vi "DAQ_Pressure_Task.vi"(8 "error in":errorcluster) -> (0 "error out":errorcluster, 3 "task out":refnum<k21>)   [LabVIEW 2015]
uses:
  <vilib>/DAQmx/configure/timing.llb/DAQmx Timing (Sample Clock).vi
  <vilib>/DAQmx/create/channels.llb/DAQmx Create Channel (AI-Current-Basic).vi
  <vilib>/DAQmx/create/channels.llb/DAQmx Create Channel (TEDS-AI-Current-Basic).vi
  <vilib>/DAQmx/create/channels.llb/DAQmx Create Channel (TEDS-AI-Voltage-Basic).vi
  <vilib>/DAQmx/create/channels.llb/DAQmx Create Channel (AI-Voltage-Basic).vi
  <resource>/objmgr/daqmx.rc
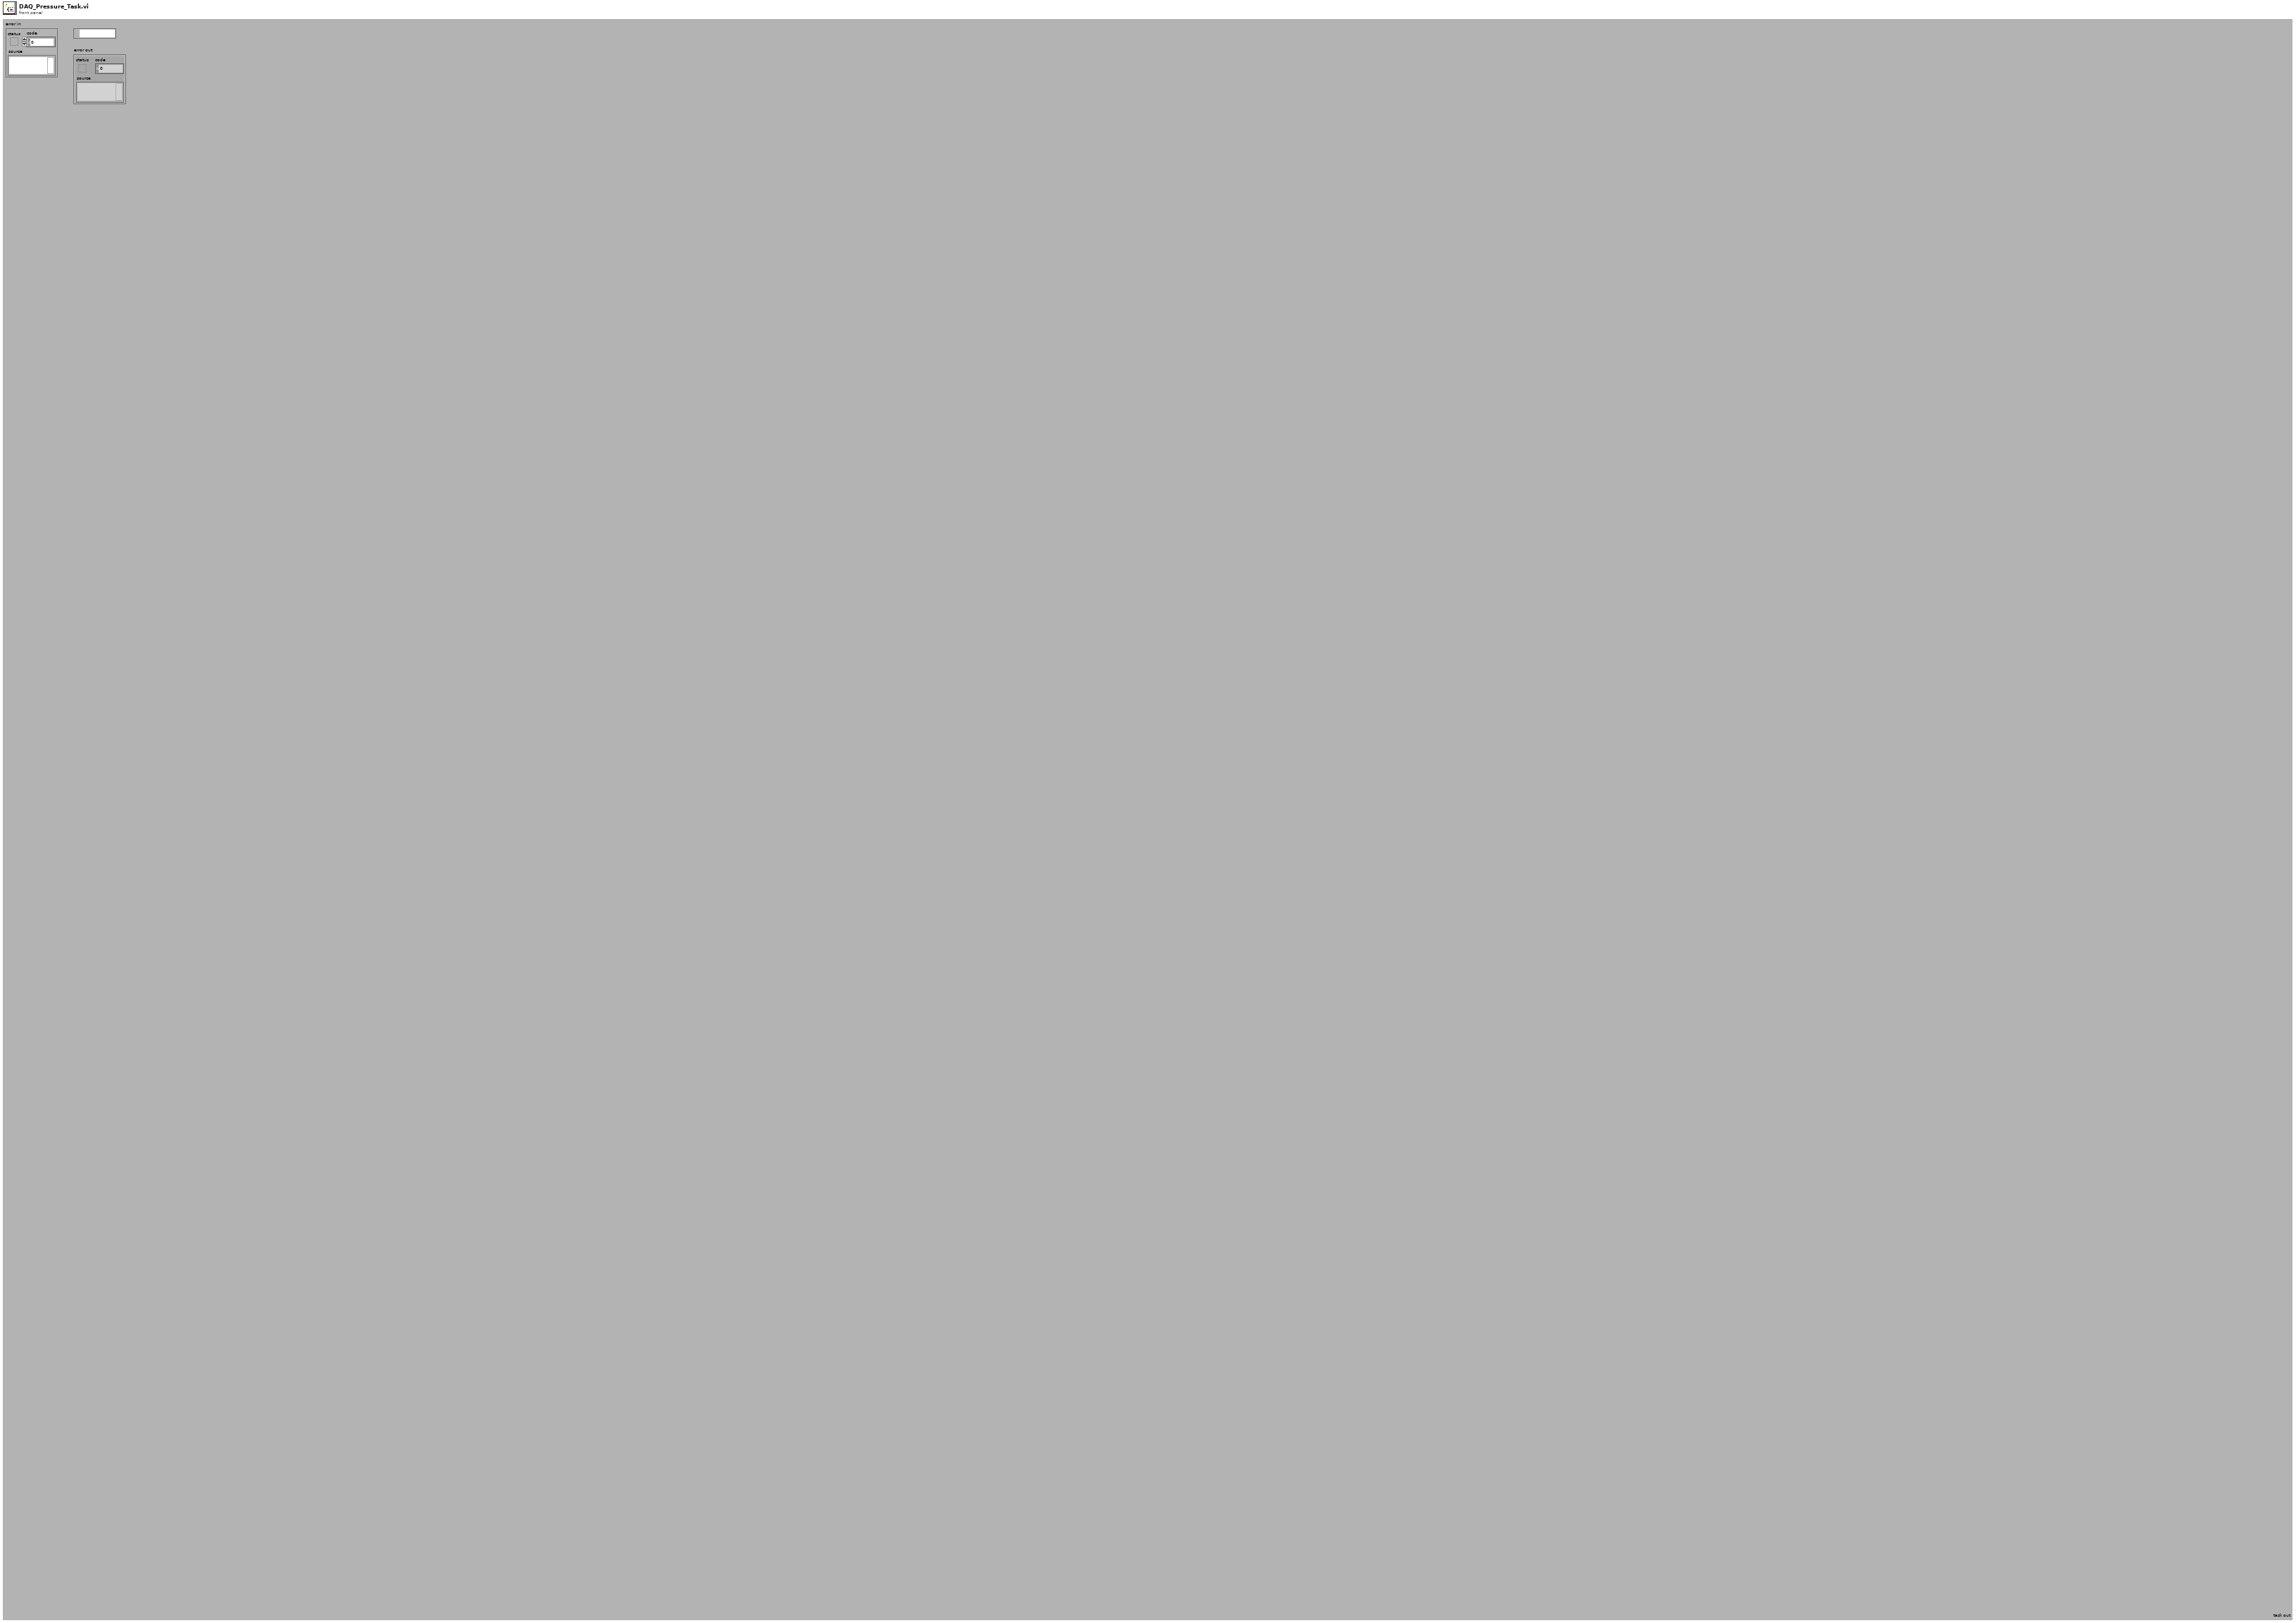
[diagram p1: front panel]
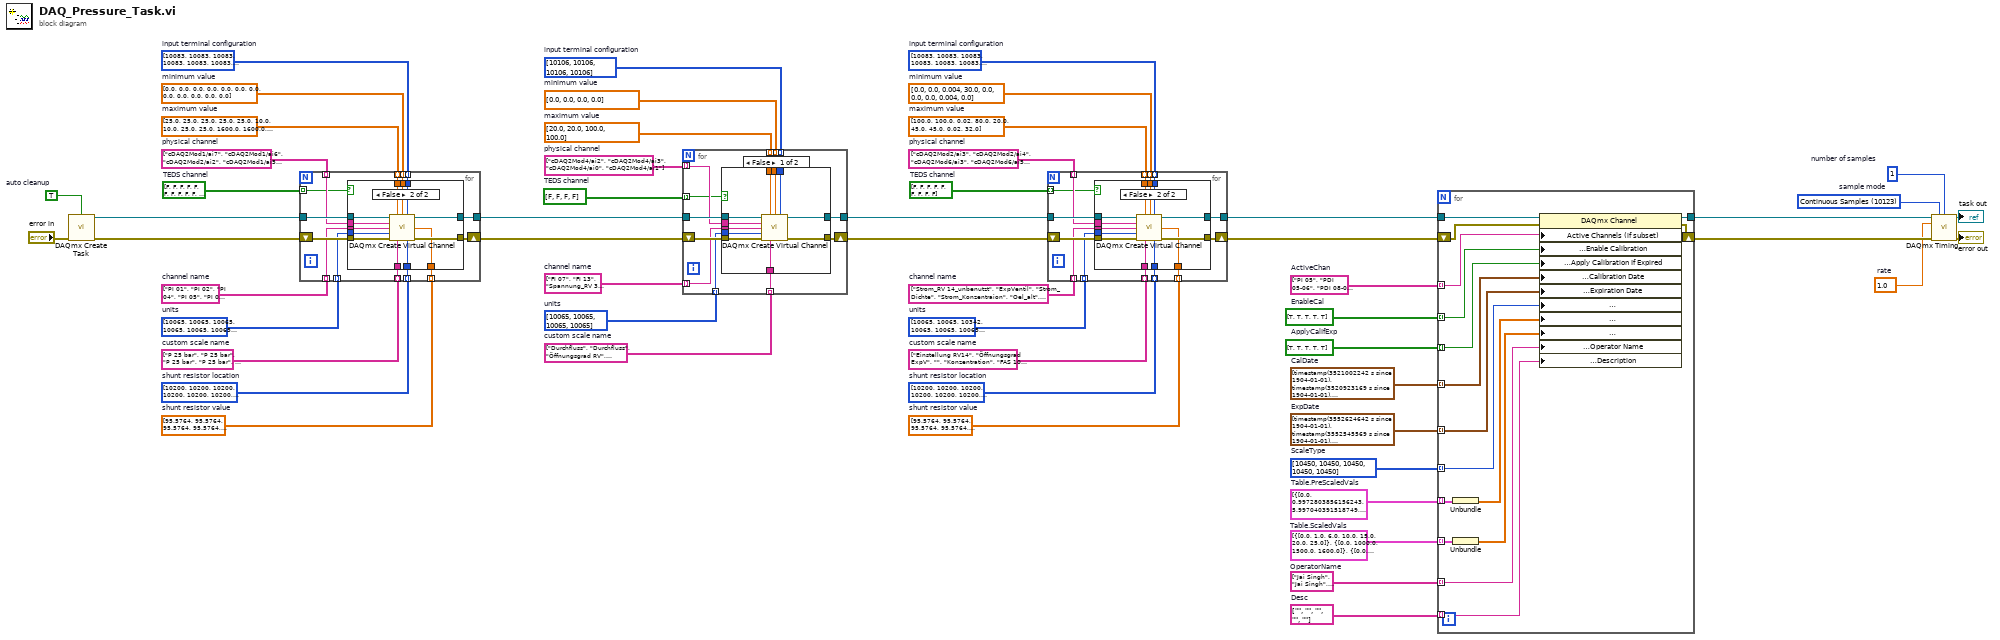
[diagram p0: block diagram]
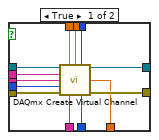
[diagram p2: hidden frame]
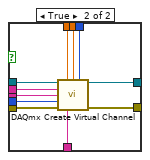
[diagram p3: hidden frame]
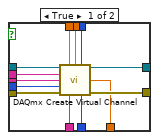
[diagram p4: hidden frame]
diagram:
  w1 = 10123 items=["Finite Samples"=10178, "Continuous Samples"=10123, "Hardware Timed Single Point"=12522]  # sample mode
  w2 = 1  # number of samples
  w3 = 1.0  # rate
  w7 = cluster{dbl[]}[] [{[0.0, 1.0, 6.0, 10.0, 15.0, 20.0, 25.0]}, {[0.0, 1000.0, 1500.0, 1600.0]}, {[0.0, 1000.0, 1500.0, 1600.0]}, {[0.0, 0.86, 1.21, 1.86, 3.1, 4.77, 6.65, 7.29, 8.84, 11.07, 13.51, 15.33, 20.0]}, {[0.004, 2.2, 3.42, 4.08, 7.7, 10.52, 12.92, 14.78, 20.74, 25.09, 26.53]}]  # Table.ScaledVals
  w8 = cluster{dbl[]}[] [{[0.0, 0.9972803856156243, 5.997040391518749, 10.015593347959374, 15.013742730296872, 20.021790629837497, 25.0]}, {[3.151240878800008, 1003.6394992132, 1504.2596451523, 1600.0]}, {[4.835925838111832, 998.5875410040248, 1496.213154230559, 1600.0]}, {[0.0, 0.6762841877287502, 1.0186559843750003, 1.6656615945525002, 2.9056125350500004, 4.562310075791251, 6.450162397260001, 7.0884341397075, 8.617806368865, 10.8448007925575, 13.286177970001251, 15.10389574293875, 20.0]}, {[0.004, 2.57, 3.6, 4.11, 7.72, 10.55, 13.02, 14.91, 21.22, 25.78, 26.53]}]  # Table.PreScaledVals
  w9 = string[] ["", "", "", "", ""]  # Desc
  w10 = string[] ["Jai Singh", "Jai Singh", "Jai Singh", "Tobi", "Max"]  # OperatorName
  w11 = timestamp[] [timestamp(3521002242.44 s since 1904-01-01), timestamp(3520923169.435 s since 1904-01-01), timestamp(3520930491.14 s since 1904-01-01), timestamp(3519973936.268 s since 1904-01-01), timestamp(3537180162.561 s since 1904-01-01)]  # CalDate
  w15 = bool[] [TRUE, TRUE, TRUE, TRUE, TRUE]  # EnableCal
  w14 = bool[] [TRUE, TRUE, TRUE, TRUE, TRUE]  # ApplyCalIfExp
  w13 = timestamp[] [timestamp(3552624642 s since 1904-01-01), timestamp(3552545569 s since 1904-01-01), timestamp(3552552891 s since 1904-01-01), timestamp(3551596336 s since 1904-01-01), timestamp(3568802563 s since 1904-01-01)]  # ExpDate
  w12 = i32[] [10450, 10450, 10450, 10450, 10450] items=["Polynomial"=10449, "Table"=10450]  # ScaleType
  w16 = string[] ["PI 05", "PDI 05-06", "PDI 08-09", "Oel_alt", "FI_Oel"]  # ActiveChan
  w19 = bool[] [FALSE, FALSE, FALSE, FALSE, FALSE, FALSE, FALSE, FALSE, FALSE]  # TEDS channel
  w21 = i32[] [10200, 10200, 10200, 10200, 10200, 10200, 10200, 10200, 10200] items=["Internal"=10200, "External"=10167]  # shunt resistor location
  w20 = dbl[] [95.5764, 95.5764, 95.5764, 95.5764, 95.5764, 95.5764, 95.5764, 95.5764, 95.5764]  # shunt resistor value
  w26 = string[] ["Einstellung RV14", "Öffnungsgrad ExpV", "", "Konzentration", "FAS 100 Öl", "FAS100 Durchfluss", "FAS100 Durchfluss", "SV5050", "Coriolis2"]  # custom scale name
  w25 = i32[] [10065, 10065, 10342, 10065, 10065, 10065, 10065, 10065, 10065] items=["Amps"=10342, "From TEDS"=12516, "From Custom Scale"=10065]  # units
  w24 = string[] ["Strom_RV 14_unbenutzt", "ExpVentil", "Strom_Dichte", "Strom_Konzentraion", "Oel_alt", "Durchfluss_FI 38", "Durchfluss_FI 35", "FI_Oel", "KaliCo"]  # channel name
  w23 = string[] ["cDAQ2Mod2/ai3", "cDAQ2Mod2/ai4", "cDAQ2Mod6/ai3", "cDAQ2Mod6/ai5", "cDAQ2Mod6/ai0", "cDAQ2Mod6/ai1", "cDAQ2Mod6/ai2", "cDAQ2Mod6/ai4", "cDAQ2Mod2/ai6"]  # physical channel
  w27 = dbl[] [100.0, 100.0, 0.02, 80.0, 20.0, 45.0, 45.0, 0.02, 32.0]  # maximum value
  w28 = dbl[] [0.0, 0.0, 0.004, 30.0, 0.0, 0.0, 0.0, 0.004, 0.0]  # minimum value
  w29 = i32[] [10083, 10083, 10083, 10083, 10083, 10083, 10083, 10083, 10083] items=["default"=-1, "RSE"=10083, "NRSE"=10078, "Differential"=10106, "Pseudodifferential"=12529]  # input terminal configuration
  w31 = bool[] [FALSE, FALSE, FALSE, FALSE]  # TEDS channel
  w36 = string[] ["Durchfluss", "Durchfluss", "Öffnungsgrad RV", "Öffnungsgrad RV"]  # custom scale name
  w35 = i32[] [10065, 10065, 10065, 10065] items=["Volts"=10348, "From TEDS"=12516, "From Custom Scale"=10065]  # units
  w34 = string[] ["FI 07", "FI 13", "Spannung_RV 39_34", "Spannung_RV 35"]  # channel name
  w33 = string[] ["cDAQ2Mod4/ai2", "cDAQ2Mod4/ai3", "cDAQ2Mod4/ai0", "cDAQ2Mod4/ai1"]  # physical channel
  w37 = dbl[] [20.0, 20.0, 100.0, 100.0]  # maximum value
  w38 = dbl[] [0.0, 0.0, 0.0, 0.0]  # minimum value
  w39 = i32[] [10106, 10106, 10106, 10106] items=["default"=-1, "RSE"=10083, "NRSE"=10078, "Differential"=10106, "Pseudodifferential"=12529]  # input terminal configuration
  w41 = bool[] [FALSE, FALSE, FALSE, FALSE, FALSE, FALSE, FALSE, FALSE, FALSE, FALSE, FALSE, FALSE]  # TEDS channel
  w43 = i32[] [10200, 10200, 10200, 10200, 10200, 10200, 10200, 10200, 10200, 10200, 10200, 10200] items=["Internal"=10200, "External"=10167]  # shunt resistor location
  w42 = dbl[] [95.5764, 95.5764, 95.5764, 95.5764, 95.5764, 95.5764, 95.5764, 95.5764, 95.5764, 95.5764, 95.5764, 95.5764]  # shunt resistor value
  w48 = string[] ["P 25 bar", "P 25 bar", "P 25 bar", "P 25 bar", "P 25 bar", "10 bar", "10 bar", "P 25 bar", "P 25 bar", "PDI-function", "PD 0-1600mbar", "Füllstand"]  # custom scale name
  w47 = i32[] [10065, 10065, 10065, 10065, 10065, 10065, 10065, 10065, 10065, 10065, 10065, 10065] items=["Amps"=10342, "From TEDS"=12516, "From Custom Scale"=10065]  # units
  w46 = string[] ["PI 01", "PI 02", "PI 04", "PI 05", "PI 07", "PI 08", "PI 11", "PI 12", "PI 14", "PDI 05-06", "PDI 08-09", "Fuellstand"]  # channel name
  w45 = string[] ["cDAQ2Mod1/ai7", "cDAQ2Mod1/ai6", "cDAQ2Mod2/ai2", "cDAQ2Mod1/ai5", "cDAQ2Mod1/ai4", "cDAQ2Mod1/ai3", "cDAQ2Mod1/ai2", "cDAQ2Mod1/ai1", "cDAQ2Mod1/ai0", "cDAQ2Mod2/ai1", "cDAQ2Mod2/ai0", "cDAQ2Mod2/ai5"]  # physical channel
  w49 = dbl[] [25.0, 25.0, 25.0, 25.0, 25.0, 10.0, 10.0, 25.0, 25.0, 1600.0, 1600.0, 1.3]  # maximum value
  w50 = dbl[] [0.0, 0.0, 0.0, 0.0, 0.0, 0.0, 0.0, 0.0, 0.0, 0.0, 0.0, 0.0]  # minimum value
  w51 = i32[] [10083, 10083, 10083, 10083, 10083, 10083, 10083, 10083, 10083, 10083, 10083, 10083] items=["default"=-1, "RSE"=10083, "NRSE"=10078, "Differential"=10106, "Pseudodifferential"=12529]  # input terminal configuration
  w53 = TRUE  # auto cleanup
  n1 = call <vilib>:"DAQmx Create Task.vi"("auto cleanup"=w53, "error in"="error in") -> ("task out"=w52:refnum<k21>, "error out"=w54:errorcluster)  [unwired: 12 in]
  n2 = for {
    tunnel: w52 -> [w66]
    tunnel: w51 -> [w69] mode=indexing
    tunnel: w50 -> [w68] mode=indexing
    tunnel: w49 -> [w67] mode=indexing
    tunnel: w48 -> [w62] mode=indexing
    tunnel: w47 -> [w59] mode=indexing
    tunnel: w46 -> [w61] mode=indexing
    tunnel: w45 -> [w60] mode=indexing
    tunnel: [w64] -> w40
    tunnel: w43 -> [w58] mode=indexing
    tunnel: w42 -> [w57] mode=indexing
    shift-right: [w63] -> w44
    shift-left: w54 -> [w65]
    tunnel: w41 -> [w56] mode=indexing
    n3 = case shown="False" w56 {
      tunnel: w69 -> [w82 w95]
      tunnel: w68 -> [w81 w94]
      tunnel: w67 -> [w80 w93]
      tunnel: w66 -> [w79 w92]
      tunnel: w65 -> [w78 w91]
      tunnel: [w77 w90] -> w64
      tunnel: [w76 w89] -> w63
      tunnel: w62 -> [w75 w88]
      tunnel: w61 -> [w74 w87]
      tunnel: w60 -> [w73 w86]
      tunnel: w59 -> [w72 w85]
      tunnel: w58 -> [w71 w84]
      tunnel: w57 -> [w70 w83]
      frame True {
        n4 = call-poly <vilib>:"DAQmx Create Virtual Channel.vi"("task in"=w79, "maximum value"=w80, "minimum value"=w81, "input terminal configuration"=w82, "physical channels"=w73, "name to assign"=w74, "external shunt resistor value"=w70, "units"=w72, "error in"=w78, "custom scale name"=w75, "shunt resistor location"=w71) -> ("task out"=w77:refnum<k21>, "error out"=w76:errorcluster)  [unwired: 3 in]
      }
      frame False {
        n5 = call-poly <vilib>:"DAQmx Create Virtual Channel.vi"("task in"=w92, "maximum value"=w93, "minimum value"=w94, "input terminal configuration"=w95, "physical channels"=w86, "name to assign"=w87, "external shunt resistor value"=w83, "units"=w85, "error in"=w91, "custom scale name"=w88, "shunt resistor location"=w84) -> ("task out"=w90:refnum<k21>, "error out"=w89:errorcluster)  [unwired: 3 in]
      }
    }
  }
  n6 = for {
    tunnel: w40 -> [w104]
    tunnel: w39 -> [w105] mode=indexing
    tunnel: w38 -> [w106] mode=indexing
    tunnel: w37 -> [w107] mode=indexing
    tunnel: w36 -> [w97] mode=indexing
    tunnel: w35 -> [w98] mode=indexing
    tunnel: w34 -> [w100] mode=indexing
    tunnel: w33 -> [w99] mode=indexing
    tunnel: [w102] -> w30
    shift-right: [w101] -> w32
    shift-left: w44 -> [w103]
    tunnel: w31 -> [w96] mode=indexing
    n7 = case shown="False" w96 {
      tunnel: w107 -> [w118 w123]
      tunnel: w106 -> [w117 w124]
      tunnel: w105 -> [w116 w125]
      tunnel: w104 -> [w115 w129]
      tunnel: w103 -> [w114 w128]
      tunnel: [w113 w126] -> w102
      tunnel: [w112 w127] -> w101
      tunnel: w100 -> [w111 w121]
      tunnel: w99 -> [w110 w122]
      tunnel: w98 -> [w109 w120]
      tunnel: w97 -> [w108 w119]
      frame False {
        n8 = call-poly <vilib>:"DAQmx Create Virtual Channel.vi"("task in"=w115, "maximum value"=w118, "minimum value"=w117, "input terminal configuration"=w116, "physical channels"=w110, "name to assign"=w111, "units"=w109, "error in"=w114, "custom scale name"=w108) -> ("task out"=w113:refnum<k21>, "error out"=w112:errorcluster)  [unwired: 5 in]
      }
      frame True {
        n9 = call-poly <vilib>:"DAQmx Create Virtual Channel.vi"("task in"=w129, "maximum value"=w123, "minimum value"=w124, "input terminal configuration"=w125, "physical channels"=w122, "name to assign"=w121, "units"=w120, "error in"=w128, "custom scale name"=w119) -> ("task out"=w126:refnum<k21>, "error out"=w127:errorcluster)  [unwired: 5 in]
      }
    }
  }
  n10 = for {
    tunnel: w30 -> [w140]
    tunnel: w29 -> [w143] mode=indexing
    tunnel: w28 -> [w142] mode=indexing
    tunnel: w27 -> [w141] mode=indexing
    tunnel: w26 -> [w136] mode=indexing
    tunnel: w25 -> [w133] mode=indexing
    tunnel: w24 -> [w135] mode=indexing
    tunnel: w23 -> [w134] mode=indexing
    tunnel: [w138] -> w18
    tunnel: w21 -> [w132] mode=indexing
    tunnel: w20 -> [w131] mode=indexing
    shift-right: [w137] -> w22
    shift-left: w32 -> [w139]
    tunnel: w19 -> [w130] mode=indexing
    n11 = case shown="False" w130 {
      tunnel: w143 -> [w156 w169]
      tunnel: w142 -> [w155 w168]
      tunnel: w141 -> [w154 w167]
      tunnel: w140 -> [w153 w166]
      tunnel: w139 -> [w152 w165]
      tunnel: [w151 w164] -> w138
      tunnel: [w150 w163] -> w137
      tunnel: w136 -> [w149 w162]
      tunnel: w135 -> [w148 w161]
      tunnel: w134 -> [w147 w160]
      tunnel: w133 -> [w146 w159]
      tunnel: w132 -> [w145 w158]
      tunnel: w131 -> [w144 w157]
      frame True {
        n12 = call-poly <vilib>:"DAQmx Create Virtual Channel.vi"("task in"=w153, "maximum value"=w154, "minimum value"=w155, "input terminal configuration"=w156, "physical channels"=w147, "name to assign"=w148, "external shunt resistor value"=w144, "units"=w146, "error in"=w152, "custom scale name"=w149, "shunt resistor location"=w145) -> ("task out"=w151:refnum<k21>, "error out"=w150:errorcluster)  [unwired: 3 in]
      }
      frame False {
        n13 = call-poly <vilib>:"DAQmx Create Virtual Channel.vi"("task in"=w166, "maximum value"=w167, "minimum value"=w168, "input terminal configuration"=w169, "physical channels"=w160, "name to assign"=w161, "external shunt resistor value"=w157, "units"=w159, "error in"=w165, "custom scale name"=w162, "shunt resistor location"=w158) -> ("task out"=w164:refnum<k21>, "error out"=w163:errorcluster)  [unwired: 3 in]
      }
    }
  }
  n14 = for {
    tunnel: w18 -> [w185]
    shift-right: [w183] -> w17
    shift-left: w22 -> [w182]
    tunnel: [w184] -> w4
    tunnel: w16 -> [w181] mode=indexing
    tunnel: w15 -> [w180] mode=indexing
    tunnel: w14 -> [w179] mode=indexing
    tunnel: w13 -> [w177] mode=indexing
    tunnel: w12 -> [w178] mode=indexing
    tunnel: w11 -> [w176] mode=indexing
    tunnel: w10 -> [w175] mode=indexing
    tunnel: w9 -> [w174] mode=indexing
    tunnel: w8 -> [w172] mode=indexing
    tunnel: w7 -> [w171] mode=indexing
    n15 = Unbundle(w172) -> (w173:dbl[])
    n16 = Unbundle(w171) -> (w170:dbl[])
    n17 = property class="DAQmx Channel"(reference=w185, error in=w182, "Active Channels (if subset)"=w181, "Analog Input:General Properties:Channel Calibration:Enable Calibration"=w180, "Analog Input:General Properties:Channel Calibration:Apply Calibration If Expired"=w179, "Analog Input:General Properties:Channel Calibration:Calibration Date"=w176, "Analog Input:General Properties:Channel Calibration:Expiration Date"=w177, "Analog Input:General Properties:Channel Calibration:Scaling Parameters:Scale Type"=w178, "Analog Input:General Properties:Channel Calibration:Scaling Parameters:Table:Pre-Scaled Values"=w173, "Analog Input:General Properties:Channel Calibration:Scaling Parameters:Table:Scaled Values"=w170, "Analog Input:General Properties:Channel Calibration:Operator Name"=w175, "Analog Input:General Properties:Channel Calibration:Description"=w174) -> (reference out=w184:refnum<k21>, error out=w183:errorcluster)
  }
  n18 = call-poly <vilib>:"DAQmx Timing.vi"("task/channels in"=w4, "sample mode"=w1, "samples per channel"=w2, "rate"=w3, "error in"=w17) -> ("task out"=→"task out":refnum<k21>, "error out"=→"error out":errorcluster)  [unwired: 9 in]
